vi "Read DER DeviceIDs.vi"(8 "error in":errorcluster, 11 "Startup Optimization in":refnum<class "Startup Optimization.lvclass">) -> (0 "error out":errorcluster, 2 "DERs":T1[](array[typedef]), 3 "Startup Optimization out":refnum<class "Startup Optimization.lvclass">)   [LabVIEW 2018, in "Startup Optimization Actor.lvlib" / "Startup Optimization.lvclass"]
uses:
  Startup Optimization.lvclass
  <vilib>/ORNL/CSEISMIC DDS/CSEISMIC DDS Base/Data Types/Controls/DeviceID.ctl
  Startup Optimization.lvclass/Startup Optimization.ctl
  <vilib>/ORNL/CSEISMIC DDS/CSEISMIC DDS Base/CSEISMIC DDS.lvclass
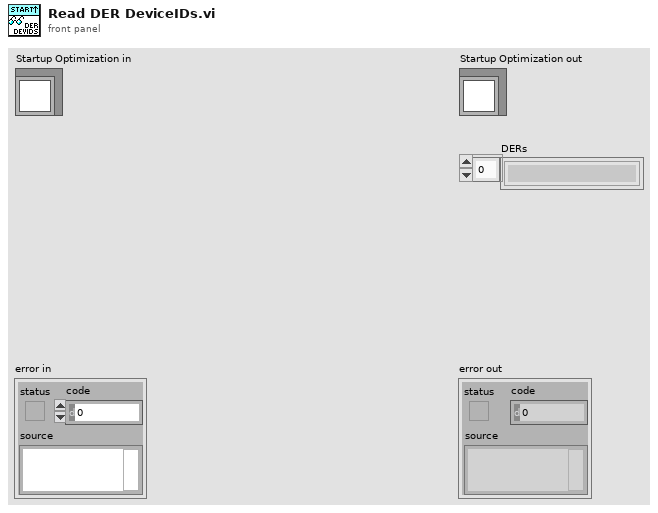
[diagram p1: front panel]
types:
  T1 = typedef "CSEISMIC DDS.lvlib/CSEISMIC DDS.lvclass/DeviceID.ctl" = string
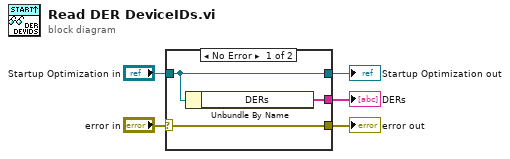
[diagram p0: block diagram]
diagram:
  n1 = case shown="No Error" "error in" {
    selector: "error in" -> [w8 w9]
    tunnel: [w8 w9] -> w4
    tunnel: [w7 w10] -> w2
    tunnel: "Startup Optimization in" -> [w7 w10]
    tunnel: [w6 _] -> w1
    frame No Error {
      n2 = Unbundle By Name(w7) -> ("DERs"=w6:T1[])
    }
    frame Error {
    }
  }
  "error out" <- w4
  "Startup Optimization out" <- w2
  "DERs" <- w1
